vi "Colonoscopy_Competition_Main.vi"() -> ()   [LabVIEW 2016]
doc: "Buggy_Competition Main.vi\nv4.0\nCode fior Jan 2012\n\nModified by D.Readman 1/12/2011 to 5/1/2012 \n- Replaced shift registers with FGV's.\n- Latched Switch function added.\n- Digital filtering on encoder inputs added."
uses:
  Controls/Plotter States.ctl
  <vilib>/Platform/TimedLoop/XDataNode/timing_clust.ctl
  <vilib>/Platform/TimedLoop/XDataNode/nitl_modes.ctl
  <vilib>/Platform/TimedLoop/XDataNode/wakeup.ctl
  <vilib>/FPGAPlugInAG/myRIO-1900/niLvFpga_Open_myRIO-1900.vi
  <vilib>/rvi/interface/nirviOpenFPGA/nirviOpenFPGA.xnode
  FPGA Bitfiles/Buggycompetition_FPGATarget2_AeroBuggyFPGA_9DbUQD1BP7s.lvbitx
  FPGA/FPGA.vi
  <vilib>/Platform/TimedLoop/XDataNode/XDataNode.xnode
  <vilib>/Platform/TimedLoop/XDataNode/XDNodeRunTimeDep.lvlib
panel:
  out "step time":dbl
  out "theoretical finish time":dbl
  out "Pot Generated Step Time":dbl
  out "total rows":i32
  out "M2 Command":dbl
  out "M1 Command":dbl
  out "row":i32
  out "current element m2":dbl
  out "motor 2 steps taken":i16
  out "motor 1 steps taken":i16
  out "current element m1":dbl
  in  "Trajectory":bool
  out "Finished Late? [i-1]":bool
  in  "Sample interval":u32=100000
  in  "MWidth":i64=4
  out "Current State":T1
  out "Switch B":bool
  out "Switch A":bool
  in  "Enc. Filter":i16=2 min=0 step=1
  out "Switches Latched":cluster{"Switch A GN":bool, "Switch B BL":bool}
  in  "Terminate":bool
  out "Error Display":errorcluster
  in  "Reset Button":bool
  # "The Classy Colonoscopy Controller"
  # "Switches"
  # "Admin controls - Do not alter"
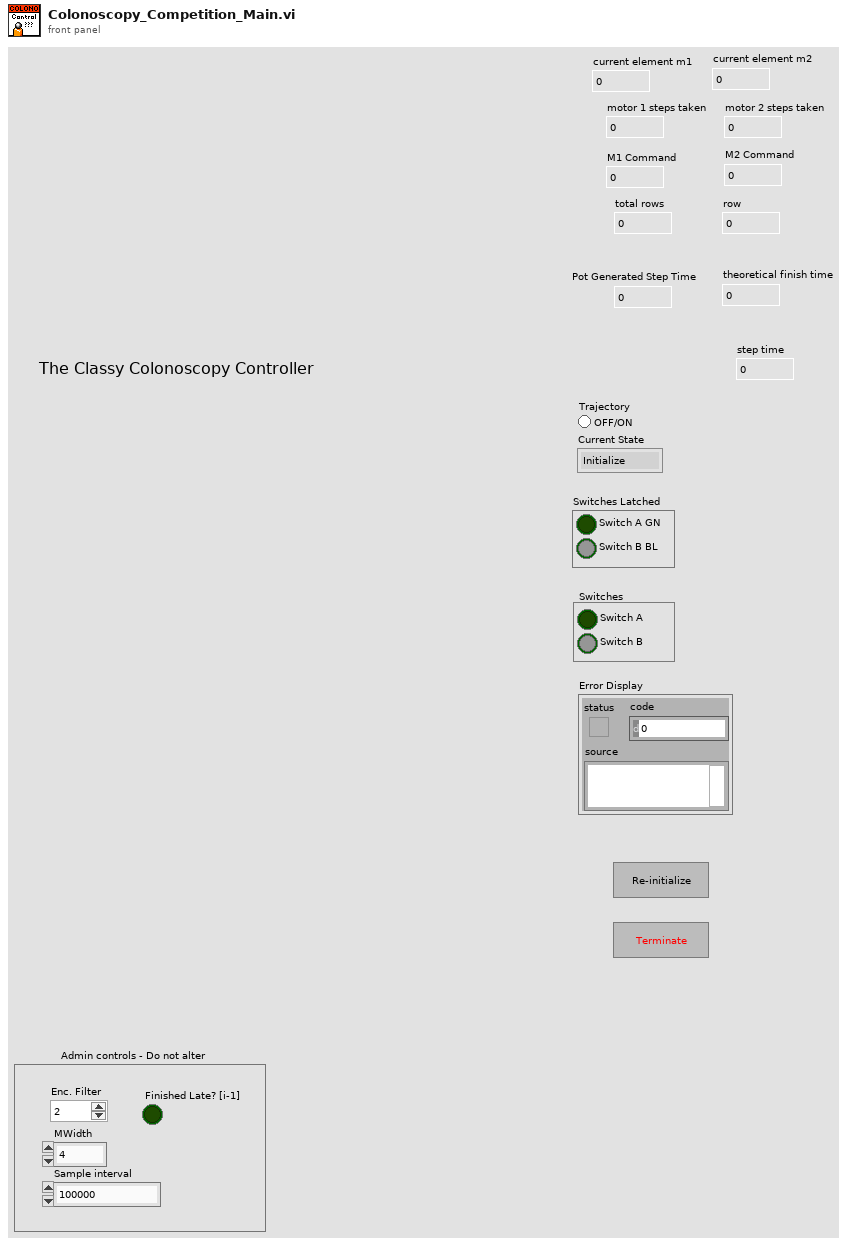
[diagram p1: front panel]
types:
  T1 = typedef "Plotter States.ctl" = enum16{"Initialize", "Run", "Stop"}
  T2 = typedef "XDNodeRunTimeDep.lvlib/timing_clust.ctl" = cluster{"Expected End [f-1]":u64, "Actual End [f-1]":u64, "Finished Late? [f-1]":bool, "Expected End [i-1]":u64, "Actual End [i-1]":u64, "Finished Late? [i-1]":bool, "Expected Start [i]":u64, "Actual Start [i]":u64, "Expected Start [f]":u64, "Actual Start [f]":u64, "Source Name":string, "Structure Name":string, "Period":i64, "Deadline":i64, "Offset":i64, "Start":i64, "Priority":i32, "Timeout":i32, "Mode":T3, "Wakeup Reason":T4, "Error":errorcluster, "Source Type":string, "Secondary Source Type":string, "Global End Time":u64, "Global Start Time":u64, "Frame Duration":u64, "Iteration Duration":u64, "Assigned CPU":i32, "I/O Scan Engine Mode":u32}
  T3 = typedef "XDNodeRunTimeDep.lvlib/nitl_modes.ctl" = enum32{"No Change", "Process missed periods, maintain original phase", "Discard missed periods, maintain original phase", "Process missed periods, ignore original phase", "Discard missed periods, ignore original phase"}
  T4 = typedef "XDNodeRunTimeDep.lvlib/wakeup.ctl" = enum32{"Normal", "Aborted", "Asynchronous wakeup", "Timing source error", "Timed loop error", "Timeout"}
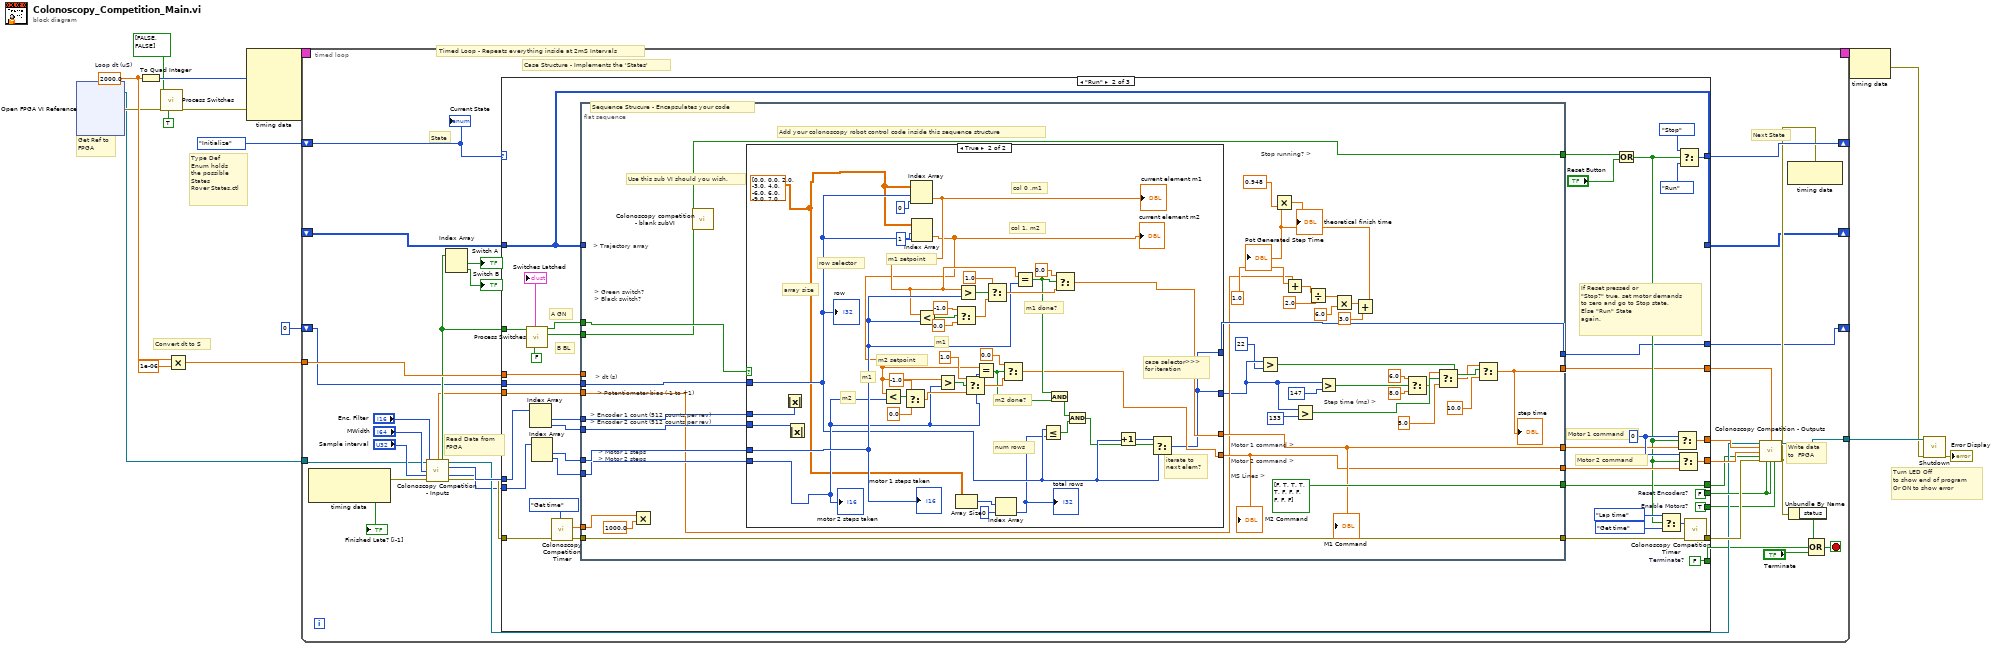
[diagram p0: block diagram]
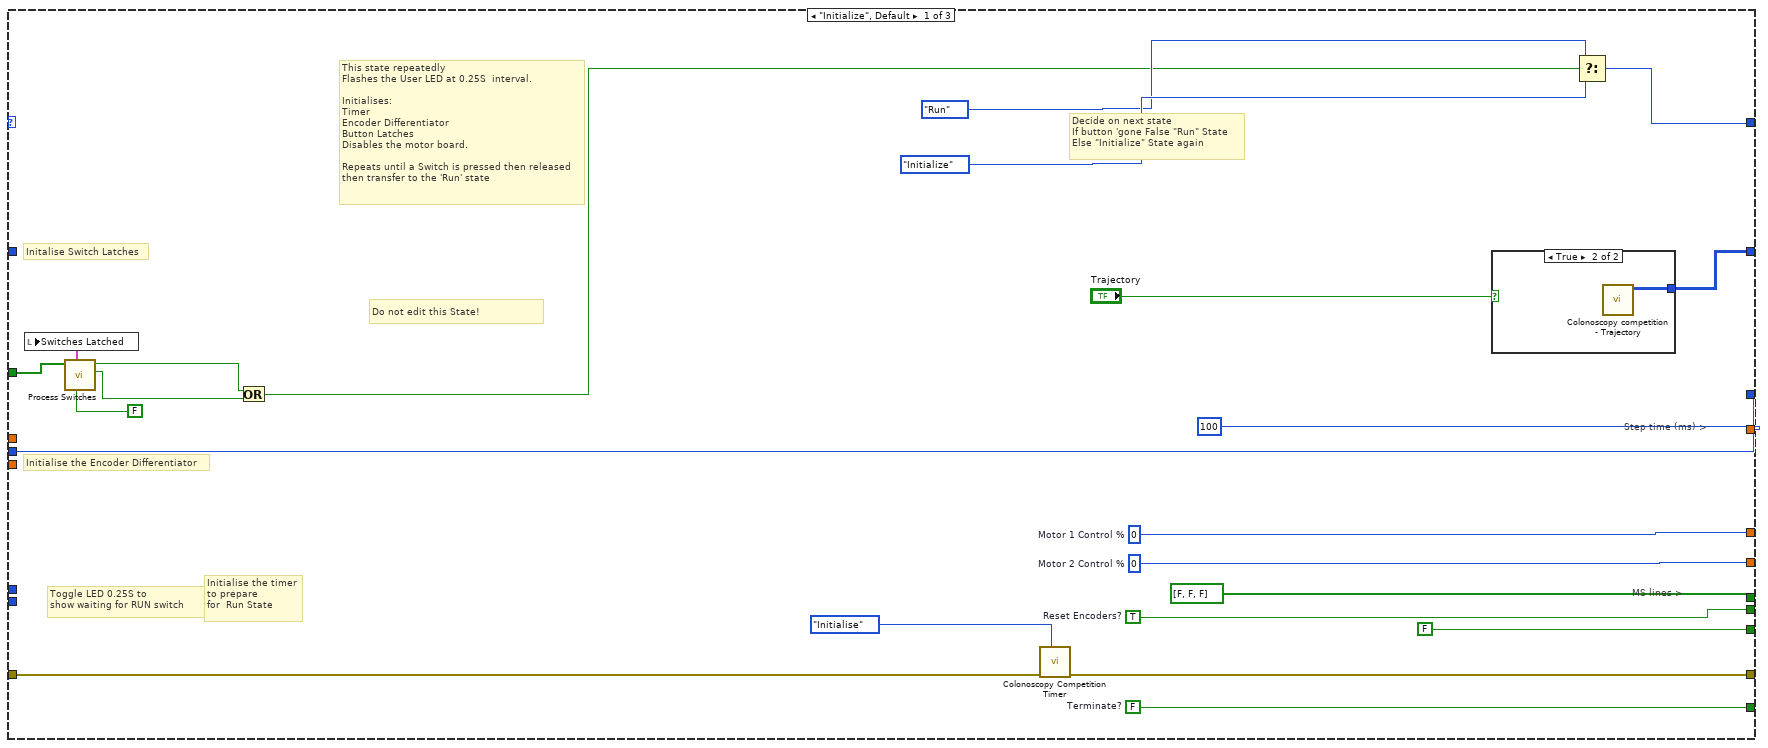
[diagram p2: hidden frame]
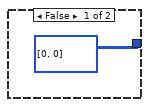
[diagram p3: hidden frame]
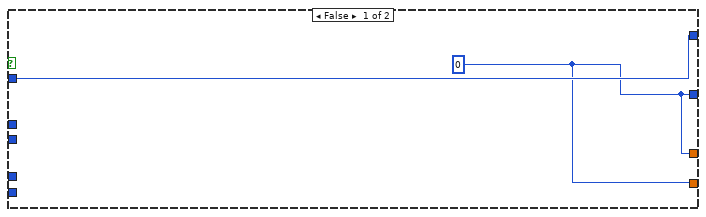
[diagram p4: hidden frame]
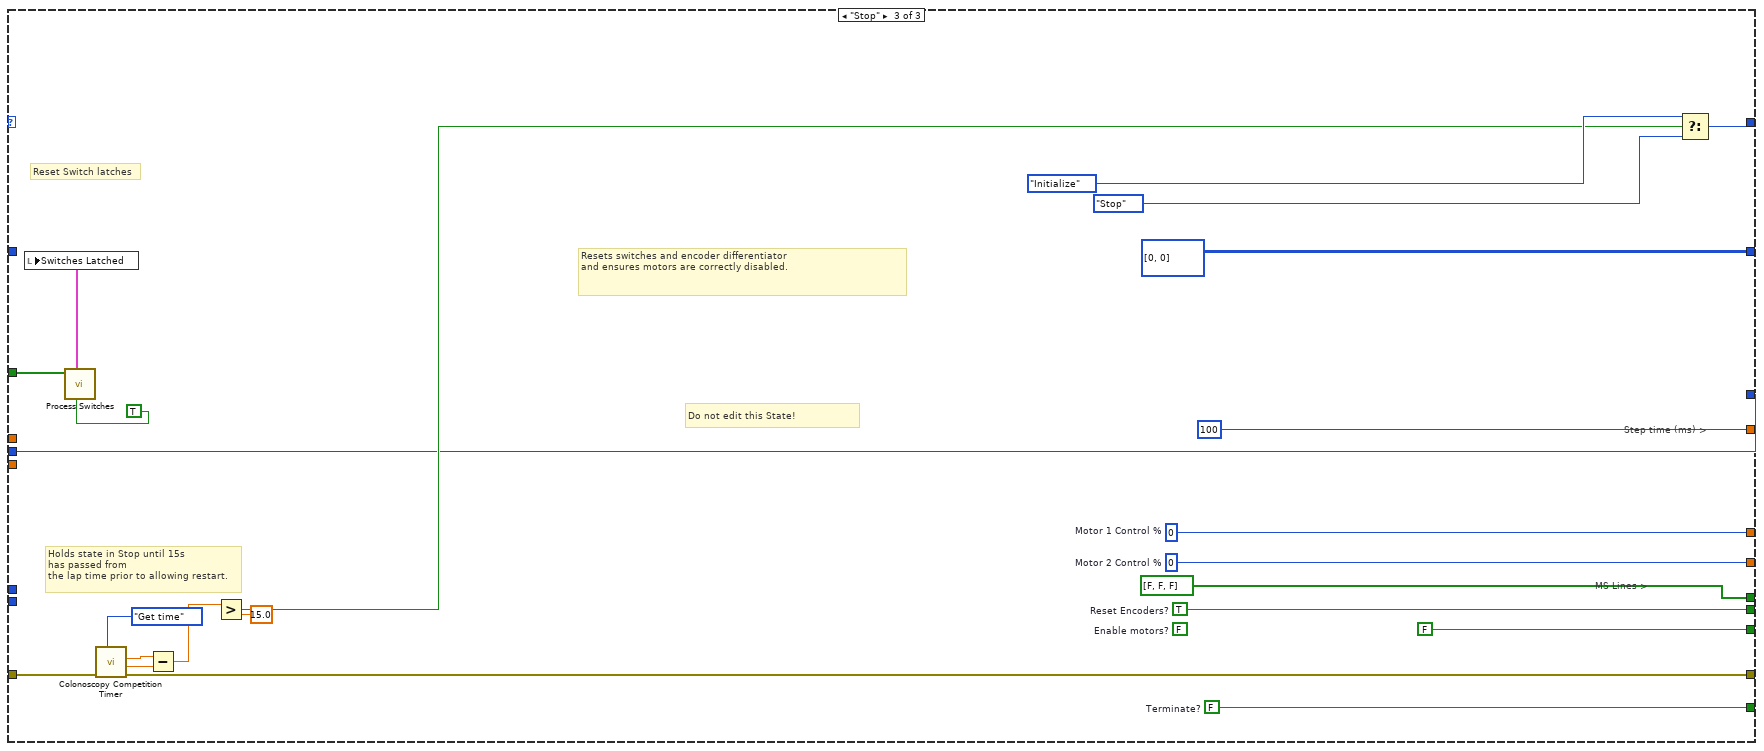
[diagram p5: hidden frame]
diagram:
  w9 = 2000.0  # Loop dt (uS)
  # "Type Def\nEnum holds\nthe possible\nStates\nRover States.ctl"
  # "Get Ref to\nFPGA"
  # "Timed Loop - Repeats everything inside at 2mS Intervals"
  # "Convert dt to S"
  # "Turn LED Off\nto show end of program\nOr ON to show error"
  n1 = xnode "Open FPGA VI Reference"() -> ("FPGA VI Reference Out"=w2:refnum<k20>, "error out"=w6:errorcluster)  [unwired: 2 in]
  n2 = To Quad Integer(1:w9) -> (0:w12:i64)
  n3 = call "Process Switches .vi"("Initialise?"=TRUE, "Error In"=w6, "Switches in"=bool[] [FALSE, FALSE]) -> ("Error Out"=w3:errorcluster)  [unwired: 4 in, 4 out]
  n4 = Multiply(x=w9, y=1e-06) -> (x*y=w7:dbl)
  n5 = node-c288(w12, w3) -> (w15:T2)  [unwired: 3 in]
  n6 = timed-loop {
    shift-right: [w49] -> _
    shift-left: Plotter_States."Initialize" ("Initial State") -> [w50]
    timing: w15 -> [_]
    timing-out: [_] -> w14
    tunnel: [w45] -> w13
    tunnel: w7 -> [w41]
    tunnel: w2 -> [w24]
    shift-right: [w21] -> _
    shift-left: _ -> [w20]
    shift-right: [w17] -> _
    shift-left: 0 -> [w18]
    stop <- w36 stop-if-true
    # "Case Structure - Implements the 'States'"
    # "Next State"
    # "Write data\nto  FPGA"
    # "Read Data from\nFPGA"
    # "State"
    n7 = node-c288() -> (w39:errorcluster, →"Finished Late? [i-1]":bool)  [unwired: 1 in]
    n8 = call "Colonoscopy Competition - Inputs.vi"("FPGA VI Reference"=w24, "Filter Iterations"="Enc. Filter", "Measurement Width (Counts)"="MWidth", "Max sample interval (uS)"="Sample interval", "Error In"=w39) -> ("Bias (-1 to +1)"=w25:dbl, "Switches Green or Black"=w27:bool[], "FPGA VI Reference Out"=w40:refnum<k20>, "Encoder count"=w48:i64[], "Motor Steps"=w30:i16[], "Error Out"=w47:errorcluster)  [unwired: 3 in, 2 out]
    n9 = Index Array(array=w27) -> (element #1=→"Switch A":bool, element #2=→"Switch B":bool)  [unwired: 2 in]
    n10 = case shown="\"Run\"" w50 {
      tunnel: [w78 w121 w216] -> w49
      tunnel: [w77 w118 w220] -> w37
      tunnel: w48 -> [_ w90 _]
      tunnel: w47 -> [w59 w84 w203]
      tunnel: [w68 w106 w205] -> w46
      tunnel: [w76 w119 w221] -> w44
      tunnel: [w75 w114 w222] -> w43
      tunnel: [w74 w113 w223] -> w42
      tunnel: w41 -> [_ w107 _]
      tunnel: w30 -> [_ w102 _]
      tunnel: w27 -> [w69 w105 w212]
      tunnel: w25 -> [_ w89 _]
      tunnel: [bool[] [FALSE, FALSE, FALSE] ("MS lines") w88 bool[] [FALSE, FALSE, FALSE] ("MS lines")] -> w23
      tunnel: [u32 100 ("Step time") w87 u32 100 ("Step time")] -> w22
      tunnel: [w64 w86 i32[][] [[0, 0]] ("Array")] -> w21
      tunnel: w20 -> [_ w86 _]
      tunnel: [FALSE ("Enable Motors?") w83 FALSE ("Enable Motors?")] -> w19
      tunnel: w18 -> [w57 w82 w201]
      tunnel: [w57 w81 w201] -> w17
      frame "Initialize", Default {
        w74 = i8 0  # Motor 2 Control %
        w75 = i8 0  # Motor 1 Control %
        w76 = TRUE  # Reset Encoders?
        w77 = FALSE  # Terminate?
        # "MS lines >"
        # "Step time (ms) >"
        # "Initalise Switch Latches"
        # "Initialise the Encoder Differentiator"
        # "This state repeatedly\nFlashes the User LED at 0.25S  interval.\n\nInitialises:\nTimer\nEncoder Differentiator\nButton Latches\nDisables the motor board.\n\nRepeats until a Switch is pressed then released\nthen transfer to the 'Run' state"
        # "Initialise the timer\nto prepare\nfor  Run State"
        # "Toggle LED 0.25S to\nshow waiting for RUN switch"
        # "Do not edit this State!"
        # "Decide on next state\nIf button 'gone False \"Run\" State\nElse \"Initialize\" State again"
        n11 = call "Process Switches .vi"("Initialise?"=FALSE, "Switches in"=w69) -> ("Switch B Latched"=w61:bool, "Switch A Latched"=w62:bool, "Switches Latched Cluster"=w72:cluster{"Switch A GN":bool, "Switch B BL":bool})  [unwired: 5 in, 2 out]
        n12 = local write "Switches Latched"(w72) -> ()
        n13 = Or(x=w62, y=w61) -> (x .or. y?=w60:bool)
        n14 = call "Colonoscopy Competition Timer.vi"("Timer state"=enum16{"Initialise", "Get time", "Lap time"}."Initialise", "Error In"=w59) -> ("Error Out"=w68:errorcluster)  [unwired: 7 in, 2 out]
        n15 = case shown="True" "Trajectory" {
          tunnel: [i32[][] [[0, 0]] ("Array") w80] -> w64
          frame False {
          }
          frame True {
            n16 = call "Colonoscopy competition - Trajectory.vi"() -> ("Array"=w80:i32[][])  [unwired: 11 in]
          }
        }
        n17 = Select(t=Plotter_States."Run" ("Buggy State"), s=w60, f=Plotter_States."Initialize" ("Buggy State")) -> (s? t:f=w78:T1)
      }
      frame "Run" {
        w112 = i8 0 ("t")
        w118 = FALSE  # Terminate?
        w83 = TRUE  # Enable Motors?
        w119 = FALSE  # Reset Encoders?
        # "If Reset pressed or\n\"Stop?\" true, set motor demands\nto zero and go to Stop state.\nElse \"Run\" State\nagain."
        # "B BL"
        # "A GN"
        # "Sequence Strucure - Encapsulates your code"
        # "Motor 2 command"
        # "Motor 1 command"
        n18 = call "Process Switches .vi"("Initialise?"=FALSE, "Switches in"=w105) -> ("Switch B Latched"=w116:bool, "Switch A Latched"=w117:bool, "Switches Latched Cluster"=→"Switches Latched":cluster{"Switch A GN":bool, "Switch B BL":bool})  [unwired: 5 in, 2 out]
        n19 = Index Array(array=w90) -> (element #1=w104:i64, element #2=w103:i64)  [unwired: 2 in]
        n20 = Index Array(array=w102) -> (element #1=w101:i16, element #2=w100:i16)  [unwired: 2 in]
        n21 = call "Colonoscopy Competition Timer.vi"("Timer state"=enum16{"Initialise", "Get time", "Lap time"}."Get time", "Error In"=w84) -> ("Error Out"=w120:errorcluster, "Elapsed Time Out (S)"=w97:dbl)  [unwired: 7 in, 1 out]
        n22 = flat-sequence {
          tunnel: [w150] -> w99
          tunnel: [w147] -> w98
          tunnel: w120 -> [w152]
          tunnel: [w152] -> w85
          tunnel: w97 -> [w158]
          tunnel: w117 -> [w159]
          tunnel: w116 -> [w151]
          tunnel: w107 -> [_]
          tunnel: w104 -> [w154]
          tunnel: w103 -> [w153]
          tunnel: w101 -> [w156]
          tunnel: w100 -> [w155]
          tunnel: [w151] -> w91
          tunnel: w89 -> [w145]
          tunnel: [bool[] [FALSE, TRUE, TRUE, TRUE, TRUE, FALSE, FALSE, FALSE, FALSE, FALSE, FALSE] ("MS lines")] -> w88
          tunnel: [w134] -> w87
          tunnel: w86 -> [_]
          tunnel: w82 -> [w149]
          tunnel: [w148] -> w81
          frame #0 {
            # "> Trajectory array"
            # "Step time (ms) >"
            # "Use this sub VI should you wish."
            # "Motor 1 command >\n\nMotor 2 command >\n\nMS Lines >"
            # "Stop running? >"
            # "> Green switch?\n> Black switch?"
            # "> dt (s)"
            # "> Potentiometer bias (-1 to +1)"
            # "> Encoder 1 count (512 counts per rev)\n> Encoder 2 count (512 counts per rev)"
            # "> Motor 1 steps\n> Motor 2 steps"
            # "Add your colonoscopy robot control code inside this sequence structure"
            n23 = Multiply(x=w158, y=1000.0 ("x*y")) -> ()  [unwired: 1 out]
            n24 = call "Colonoscopy competition - blank subVI.vi"() -> ()  [unwired: 12 in, 4 out]
            n25 = case shown="True" w159 {
              tunnel: w156 -> [_ w187]
              tunnel: w155 -> [_ w178]
              tunnel: w154 -> [_ w200]
              tunnel: w153 -> [_ w199]
              tunnel: [w161 w168] -> w150
              tunnel: w149 -> [w162 w173]
              tunnel: [w162 w163] -> w148
              tunnel: [w161 w169] -> w147
              tunnel: [w161 w163] -> w127
              frame False {
                w161 = 0
              }
              frame True {
                w164 = dbl[][] [[0.0, 0.0], [2.0, -3.0], [4.0, -6.0], [6.0, -9.0], [7.0, -11.0], [8.0, -12.0], [10.0, -15.0], [12.0, -17.0], [13.0, -19.0], [15.0, -21.0], [17.0, -23.0], [19.0, -24.0], [23.0, -22.0], [26.0, -19.0], [30.0, -14.0], [33.0, -9.0], [37.0, -2.0], [42.0, 6.0], [44.0, 9.0], [46.0, 12.0], [51.0, 17.0], [58.0, 25.0], [65.0, 32.0], [69.0, 36.0], [73.0, 40.0], [78.0, 46.0], [82.0, 48.0], [85.0, 51.0], [90.0, 55.0], [93.0, 56.0], [96.0, 58.0], [99.0, 59.0], [102.0, 60.0], [107.0, 61.0], [111.0, 61.0], [114.0, 61.0], [116.0, 61.0], [118.0, 60.0], [120.0, 59.0], [122.0, 58.0], [124.0, 57.0], [126.0, 56.0], [128.0, 55.0], [131.0, 52.0], [133.0, 49.0], [135.0, 46.0], [137.0, 44.0], [139.0, 40.0], [141.0, 37.0], [142.0, 35.0], [143.0, 33.0], [144.0, 29.0], [145.0, 27.0], [146.0, 24.0], [147.0, 20.0], [148.0, 16.0], [149.0, 13.0], [149.0, 10.0], [150.0, 8.0], [150.0, 5.0], [151.0, 3.0], [152.0, -1.0], [153.0, -5.0], [154.0, -9.0], [155.0, -12.0], [156.0, -16.0], [158.0, -19.0], [159.0, -21.0], [160.0, -24.0], [161.0, -26.0], [162.0, -29.0], [163.0, -31.0], [165.0, -35.0], [167.0, -38.0], [169.0, -41.0], [170.0, -44.0], [172.0, -47.0], [174.0, -51.0], [177.0, -54.0], [178.0, -56.0], [181.0, -60.0], [184.0, -64.0], [186.0, -67.0], [188.0, -69.0], [189.0, -72.0], [190.0, -76.0], [190.0, -80.0], [189.0, -83.0], [186.0, -86.0], [182.0, -88.0], [180.0, -88.0], [177.0, -89.0], [174.0, -89.0], [171.0, -89.0], [168.0, -89.0], [165.0, -90.0], [161.0, -90.0], [157.0, -91.0], [153.0, -92.0], [150.0, -92.0], [148.0, -93.0], [143.0, -94.0], [140.0, -95.0], [137.0, -96.0], [134.0, -97.0], [130.0, -98.0], [126.0, -99.0], [124.0, -100.0], [122.0, -101.0], [118.0, -103.0], [115.0, -105.0], [113.0, -107.0], [111.0, -108.0], [108.0, -110.0], [105.0, -112.0], [102.0, -115.0], [101.0, -117.0], [99.0, -119.0], [96.0, -122.0], [95.0, -124.0], [94.0, -125.0], [91.0, -129.0], [89.0, -132.0], [87.0, -136.0], [87.0, -138.0], [85.0, -141.0], [84.0, -144.0], [83.0, -148.0], [81.0, -150.0], [81.0, -153.0], [80.0, -156.0], [79.0, -158.0], [78.0, -161.0], [77.0, -163.0], [76.0, -167.0], [75.0, -171.0], [75.0, -174.0], [74.0, -177.0], [74.0, -180.0], [73.0, -185.0], [72.0, -189.0], [72.0, -191.0], [72.0, -196.0], [71.0, -200.0], [70.0, -204.0], [67.0, -206.0], [63.0, -206.0], [60.0, -204.0], [58.0, -202.0], [54.0, -199.0], [51.0, -196.0], [47.0, -193.0], [44.0, -190.0], [41.0, -188.0], [38.0, -186.0], [35.0, -184.0], [32.0, -182.0], [30.0, -180.0], [27.0, -178.0], [25.0, -177.0], [22.0, -175.0], [20.0, -174.0], [18.0, -173.0], [16.0, -171.0], [14.0, -170.0], [12.0, -169.0], [8.0, -167.0], [4.0, -165.0], [0.0, -164.0], [-3.0, -162.0], [-6.0, -161.0], [-9.0, -160.0], [-12.0, -159.0], [-14.0, -158.0], [-17.0, -157.0], [-19.0, -157.0], [-21.0, -156.0], [-25.0, -155.0], [-29.0, -154.0], [-32.0, -153.0], [-35.0, -153.0], [-38.0, -152.0], [-43.0, -151.0], [-46.0, -151.0], [-49.0, -150.0], [-53.0, -150.0], [-57.0, -149.0], [-61.0, -148.0], [-63.0, -146.0], [-63.0, -143.0], [-62.0, -140.0], [-60.0, -137.0], [-57.0, -132.0], [-54.0, -128.0], [-49.0, -123.0], [-44.0, -120.0], [-39.0, -118.0], [-35.0, -116.0], [-30.0, -113.0], [-24.0, -111.0], [-21.0, -109.0], [-19.0, -107.0], [-15.0, -105.0], [-10.0, -101.0], [-5.0, -97.0], [-1.0, -93.0], [1.0, -89.0], [2.0, -86.0], [3.0, -84.0], [3.0, -82.0], [3.0, -78.0], [3.0, -74.0], [3.0, -72.0], [4.0, -68.0], [4.0, -65.0], [6.0, -62.0], [8.0, -59.0], [10.0, -57.0], [14.0, -55.0], [19.0, -54.0], [22.0, -53.0], [25.0, -53.0], [28.0, -53.0], [33.0, -52.0], [36.0, -52.0], [39.0, -52.0], [42.0, -51.0], [46.0, -51.0], [48.0, -53.0], [49.0, -55.0], [50.0, -56.0], [52.0, -59.0], [54.0, -60.0], [55.0, -62.0], [57.0, -64.0], [59.0, -66.0], [59.0, -66.0]] ("all rows")
                # "array size"
                # "m1 setpoint"
                # "m1"
                # "m2 setpoint"
                # "num rows"
                # "m2"
                # "m1"
                # "m1 done?"
                # "case selector>>>\nfor iteration"
                # "m2 done?"
                # "row selector"
                # "col 1, m2"
                # "col 0 ,m1"
                # "iterate to next elem?"
                n26 = Absolute Value(x=w200) -> ()  [unwired: 1 out]
                n27 = Absolute Value(x=w199) -> ()  [unwired: 1 out]
                n28 = Index Array(array=w164, index (row)=w173, index (col)=0 ("disabled index (col)")) -> (element=w186:dbl)
                "current element m1" <- w186
                n29 = Index Array(array=w164, index (row)=w173, index (col)=1 ("disabled index (col)")) -> (element=w176:dbl)
                "current element m2" <- w176
                n30 = Less?(x=w176, y=w178) -> (x < y?=w184:bool)
                n31 = Select(t=-1.0, s=w184, f=0.0) -> (s? t:f=w185:dbl)
                n32 = Less?(x=w186, y=w187) -> (x < y?=w190:bool)
                n33 = Greater?(x=w176, y=w178) -> (0:w177:bool)
                n34 = Select(t=-1.0, s=w190, f=0.0) -> (s? t:f=w193:dbl)
                n35 = Array Size(array=w164) -> (size(s)=w167:i32[])
                n36 = Greater?(x=w186, y=w187) -> (0:w195:bool)
                n37 = Select(t=1.0, s=w177, f=w185) -> (s? t:f=w181:dbl)
                n38 = Equal?(x=w176, y=w178) -> (x = y?=w174:bool)
                n39 = Select(t=1.0, s=w195, f=w193) -> (s? t:f=w191:dbl)
                n40 = Index Array(array=w167, index=0) -> (element=w165:i32)
                "total rows" <- w165
                n41 = Select(t=0.0, s=w174, f=w181) -> (s? t:f=w169:dbl)
                n42 = Equal?(x=w186, y=w187) -> (x = y?=w175:bool)
                n43 = Less Or Equal?(x=w173, y=w165) -> (x <= y?=w171:bool)
                n44 = And(x=w175, y=w174) -> (x .and. y?=w172:bool)
                n45 = Select(t=0.0, s=w175, f=w191) -> (s? t:f=w168:dbl)
                n46 = And(x=w172, y=w171) -> (x .and. y?=w170:bool)
                n47 = Increment(x=w173) -> (x+1=w196:i32)
                n48 = Select(t=w196, s=w170, f=w173) -> (s? t:f=w163:i32)
                "motor 1 steps taken" <- w187
                "motor 2 steps taken" <- w178
                "row" <- w173
              }
            }
            "M1 Command" <- w150
            "M2 Command" <- w147
            n49 = Greater?(x=w127, y=22) -> (0:w135:bool)
            n50 = Add(x=1.0, y=w145) -> (x+y=w144:dbl)
            n51 = Greater?(x=w127, y=133) -> (0:w132:bool)
            n52 = Divide(x=w144, y=2.0) -> (x/y=w142:dbl)
            n53 = Greater?(x=w127, y=147) -> (0:w131:bool)
            n54 = Multiply(x=w142, y=6.0) -> (x*y=w140:dbl)
            n55 = Add(x=w140, y=3.0) -> (x+y=w138:dbl)
            "Pot Generated Step Time" <- w138
            n56 = Multiply(x=w138, y=0.948) -> (x*y=→"theoretical finish time":dbl)
            n57 = Select(t=6.0, s=w131, f=8.0) -> (s? t:f=w124:dbl)
            n58 = Select(t=w124, s=w132, f=5.0 ("t")) -> (s? t:f=w122:dbl)
            n59 = Select(t=w122, s=w135, f=10.0) -> (s? t:f=w134:dbl)
            "step time" <- w134
          }
        }
        n60 = Or(x=w91, y="Reset Button") -> (x .or. y?=w93:bool)
        n61 = Select(t=enum16{"Initialise", "Get time", "Lap time"}."Lap time" ("Timer state"), s=w93, f=enum16{"Initialise", "Get time", "Lap time"}."Get time" ("Timer state")) -> (s? t:f=w95:enum16{"Initialise", "Get time", "Lap time"})
        n62 = Select(t=w112, s=w93, f=w99) -> (s? t:f=w114:dbl)
        n63 = Select(t=w112, s=w93, f=w98) -> (s? t:f=w113:dbl)
        n64 = Select(t=Plotter_States."Stop" ("Buggy State"), s=w93, f=Plotter_States."Run" ("Buggy State")) -> (s? t:f=w121:T1)
        n65 = call "Colonoscopy Competition Timer.vi"("Timer state"=w95, "Error In"=w85) -> ("Error Out"=w106:errorcluster)  [unwired: 7 in, 2 out]
      }
      frame "Stop" {
        w220 = FALSE  # Terminate?
        (unwired) FALSE  # Enable motors?
        w221 = TRUE  # Reset Encoders?
        w222 = i8 0  # Motor 1 Control %
        w223 = i8 0  # Motor 2 Control %
        # "MS Lines >"
        # "Step time (ms) >"
        # "Holds state in Stop until 15s\nhas passed from\nthe lap time prior to allowing restart."
        # "Resets switches and encoder differentiator\nand ensures motors are correctly disabled."
        # "Do not edit this State!"
        # "Reset Switch latches"
        n66 = call "Process Switches .vi"("Initialise?"=TRUE, "Switches in"=w212) -> ("Switches Latched Cluster"=w218:cluster{"Switch A GN":bool, "Switch B BL":bool})  [unwired: 5 in, 4 out]
        n67 = local write "Switches Latched"(w218) -> ()
        n68 = call "Colonoscopy Competition Timer.vi"("Timer state"=enum16{"Initialise", "Get time", "Lap time"}."Get time", "Error In"=w203) -> ("Error Out"=w205:errorcluster, "Lap time out (s)"=w210:dbl, "Elapsed Time Out (S)"=w209:dbl)  [unwired: 7 in]
        n69 = Subtract(x=w209, y=w210) -> (x-y=w204:dbl)
        n70 = Greater?(x=w204, y=15.0) -> (0:w213:bool)
        n71 = Select(t=Plotter_States."Initialize" ("Buggy State"), s=w213, f=Plotter_States."Stop") -> (s? t:f=w216:T1)
      }
    }
    n72 = call "Colonoscopy Competition - Outputs.vi"("FPGA VI Reference"=w40, "Step time"=w22, "Motor 1 command"=w43, "Motor 2 command"=w42, "MS lines"=w23, "Error In"=w46, "Reset encoder 1?"=w44, "Reset encoder 2?"=w44, "Enable motors?"=w19) -> ("FPGA VI Reference out"=w45:refnum<k20>, "Error Out"=w34:errorcluster)  [unwired: 5 in]
    n73 = node-c288(w34) -> ()  [unwired: 1 out]
    n74 = Unbundle By Name(w34) -> ("status"=w38:bool)
    n75 = Compound Arithmetic op=OR(w38, w37, "Terminate") -> (w36:bool)
    "Current State" <- w50
  }
  n76 = node-c288(w14) -> (w11:errorcluster)
  n77 = call "Shutdown.vi"("Error"=w11, "FPGA VI Reference"=w13) -> ("Error Display"=→"Error Display":errorcluster)  [unwired: 8 in]
